vi "Write args.vi"(8 "error in":errorcluster, 10 "args":string[](array[string]), 11 "Shared Library Module configuration in":refnum<class "Shared Library Module configuration.lvclass">) -> (0 "error out":errorcluster, 3 "Shared Library Module configuration out":refnum<class "Shared Library Module configuration.lvclass">)   [LabVIEW 2013, in "Shared Library Module configuration.lvclass"]
uses:
  Shared Library Module configuration.lvclass
  Shared Library Module configuration.lvclass/Shared Library Module configuration.ctl
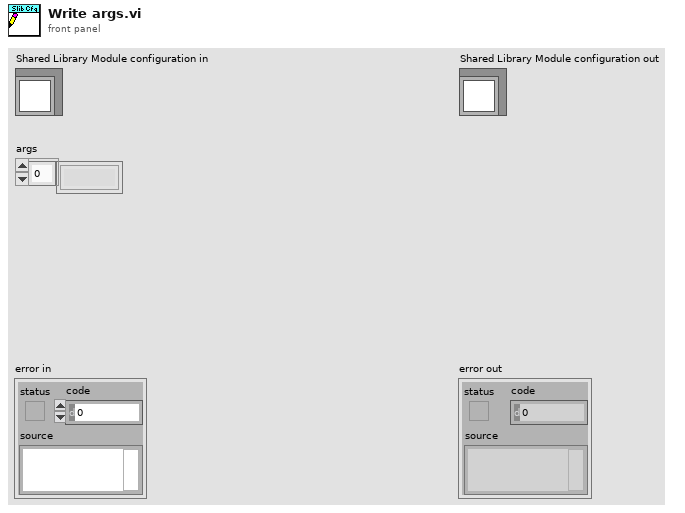
[diagram p1: front panel]
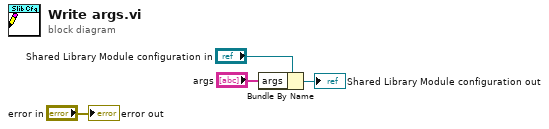
[diagram p0: block diagram]
diagram:
  n1 = Bundle By Name(cluster="Shared Library Module configuration in", "args"="args") -> (→"Shared Library Module configuration out":refnum<class "Shared Library Module configuration.lvclass">)
  "error out" <- "error in"
